vi "Gaussian.vi"(6 "STEPS":i32, 9 "POSITION":i32, 10 "y":dbl[](array[numeric]), 11 "x":dbl[](array[numeric])) -> (3 "Gaussian":dbl[](array[numeric]))   [LabVIEW 2019]
panel:
  out "Dev standard":dbl
  out "Average":dbl
  out "Interferogram":cluster{"Array":dbl[], "Array":dbl[]}(graph)
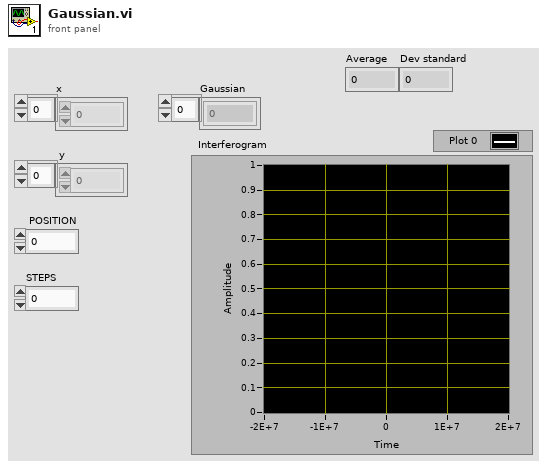
[diagram p1: front panel]
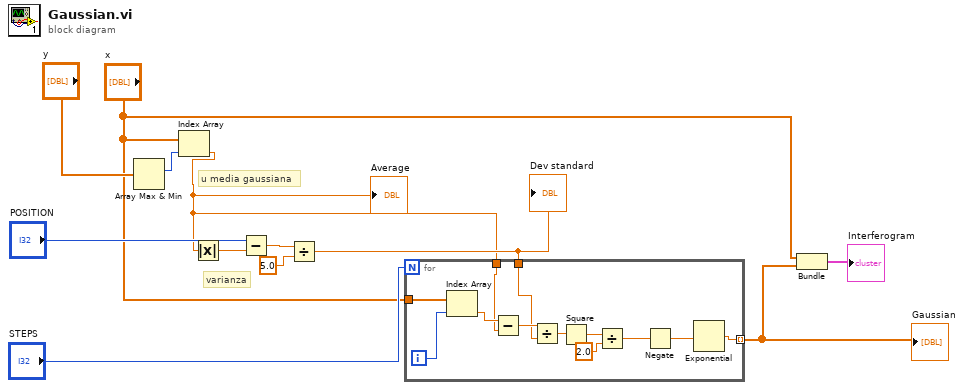
[diagram p0: block diagram]
diagram:
  # "varianza"
  # "u media gaussiana"
  n1 = Array Max & Min(array="y") -> (max index (indices)=w6:i32)  [unwired: 3 out]
  n2 = Index Array(array="x", index=w6) -> (element=w1:dbl)
  "Average" <- w1
  n3 = Absolute Value(x=w1) -> (abs(x)=w8:dbl)
  n4 = Subtract(x="POSITION", y=w8) -> (x-y=w9:dbl)
  n5 = Divide(x=w9, y=5.0) -> (x/y=w12:dbl)
  "Dev standard" <- w12
  n6 = for {
    N: "STEPS" -> [_]
    tunnel: "x" -> [w24]
    tunnel: w1 -> [w21]
    tunnel: w12 -> [w19]
    tunnel: [w15] -> w3 mode=indexing
    i -> [w23]
    n7 = Index Array(array=w24, index=w23) -> (element=w22:dbl)
    n8 = Subtract(x=w22, y=w21) -> (x-y=w20:dbl)
    n9 = Divide(x=w20, y=w19) -> (x/y=w18:dbl)
    n10 = Square(x=w18) -> (x^2=w17:dbl)
    n11 = Divide(x=w17, y=2.0) -> (x/y=w13:dbl)
    n12 = Negate(x=w13) -> (-x=w14:dbl)
    n13 = Exponential(1:w14) -> (0:w15:dbl)
  }
  "Gaussian" <- w3
  n14 = Bundle("x"="x", w3) -> (→"Interferogram":cluster{"x":dbl[], dbl[]})  [unwired: 1 in]
